vi "Email_notification.vi"(0 "Email":string) -> ()   [LabVIEW 2016]
uses:
  Global/Global Variables/Data_Display_global.vi
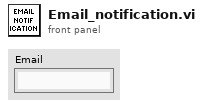
[diagram p1: front panel]
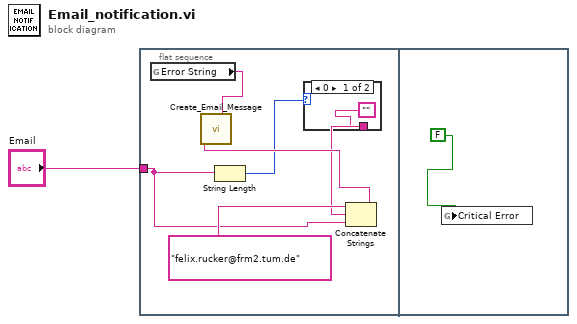
[diagram p0: block diagram]
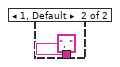
[diagram p2: hidden frame]
diagram:
  n1 = flat-sequence {
    tunnel: "Email" -> [w2]
    frame #0 {
      n2 = global read "Data_Display_global.vi" "Error String"() -> (w3:string)
      n3 = String Length(string=w2) -> (length=w5:i32)
      n4 = case shown="0" w5 {
        tunnel: ["" ", "] -> w4
        frame 0 {
        }
        frame 1, Default {
        }
      }
      n5 = Concatenate Strings("felix.rucker@frm2.tum.de", w4, w2) -> (w6:string)
      n6 = call "Create_Email_Message.vi"("Responsible Mail"=w6, "Warning"=w3) -> ()  [unwired: 10 in]
    }
    frame #1 {
      n7 = global write "Data_Display_global.vi" "Critical Error"(FALSE) -> ()
    }
  }
